vi "Check Tag WarnNSEstop Threshold.vi"(0 "Tick Counts Since Last Over Threshold":T4(array[cluster]), 1 "Warn/NS/Estop (0/1/2)":i32, 5 "Current Tick Count":u32, 7 "Tag from APU Setup File":string, 9 "Row of Tag/Warn/NS/Estop Vals":dbl[](array[numeric]), 11 "error in (no error)":errorcluster, 12 "Parsed Tags in":T2, 13 "Threshold Type (Neither/Max/Min)":enum16{"Neither", "Max", "Min"}(ring)) -> (4 "Tick Counts Since Last Over Threshold out":T4(array[cluster]), 8 "Alert":bool, 10 "Tag Thresh Info":T1, 15 "error out":errorcluster)   [LabVIEW 2018, in "RT - Analysis.lvlib"]
uses:
  RT - Analysis.lvlib
  Private Controls/Parsed Data Arrays.ctl
  Top Level/Shared Controls/Parsed Tag Cluster.ctl
  Public Controls/Alert Data.ctl
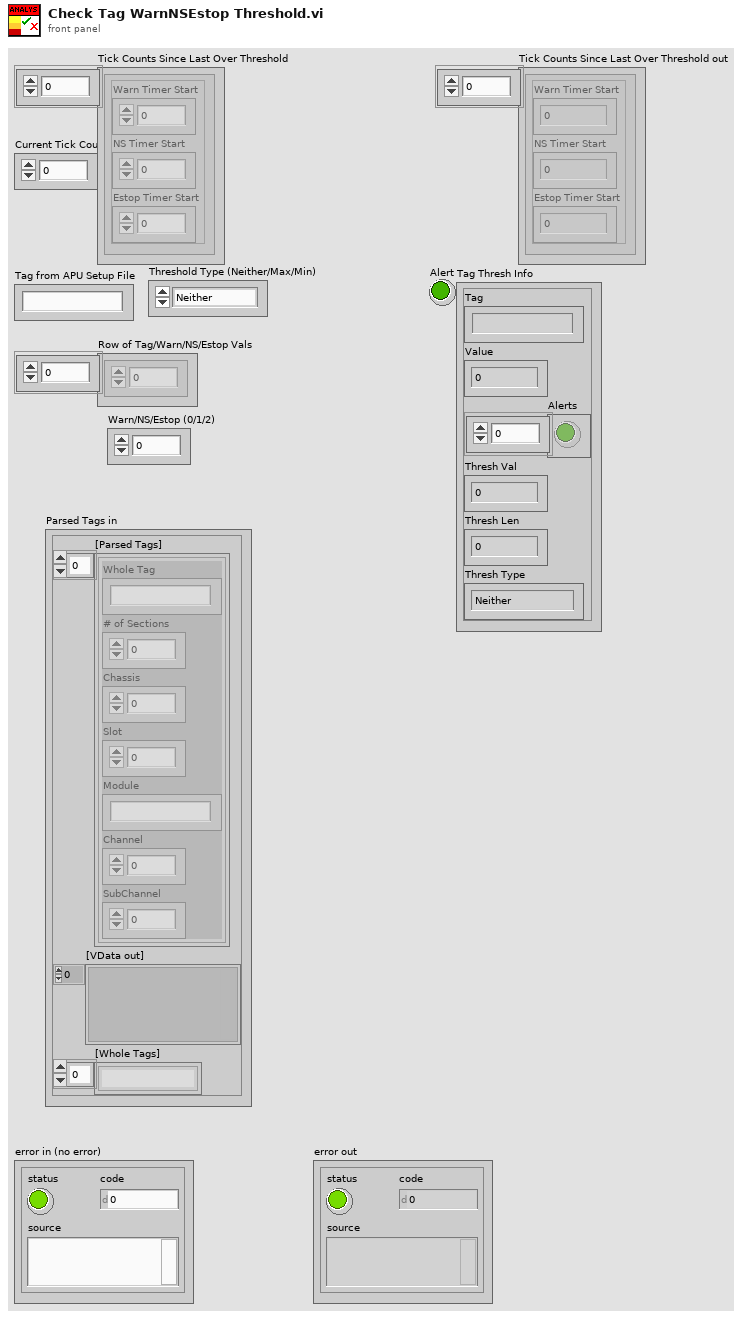
[diagram p1: front panel]
types:
  T1 = typedef "RT - Analysis.lvlib/Alert Data.ctl" = cluster{"Tag":string, "Value":dbl, "Alerts":bool[], "Thresh Val":dbl, "Thresh Len":dbl, "Thresh Type":enum16{"Neither", "Max", "Min"}}
  T2 = typedef "RT - Analysis.lvlib/Parsed Data Arrays.ctl" = cluster{"[Parsed Tags]":T3[], "[VData out]":variant[], "[Whole Tags]":string[]}
  T3 = typedef "Parsed Tag Cluster.ctl" = cluster{"Whole Tag":string, "# of Sections":u8, "Chassis":u8, "Slot":u8, "Module":string, "Channel":u8, "SubChannel":u8}
  T4 = cluster{"Warn Timer Start":u32, "NS Timer Start":u32, "Estop Timer Start":u32}[]
  T5 = cluster{"Warn Timer Start":u32, "NS Timer Start":u32, "Estop Timer Start":u32}
  T6 = cluster{"Warn Timer Start":u32, "Warn Timer Start":u32, "Warn Timer Start":u32}
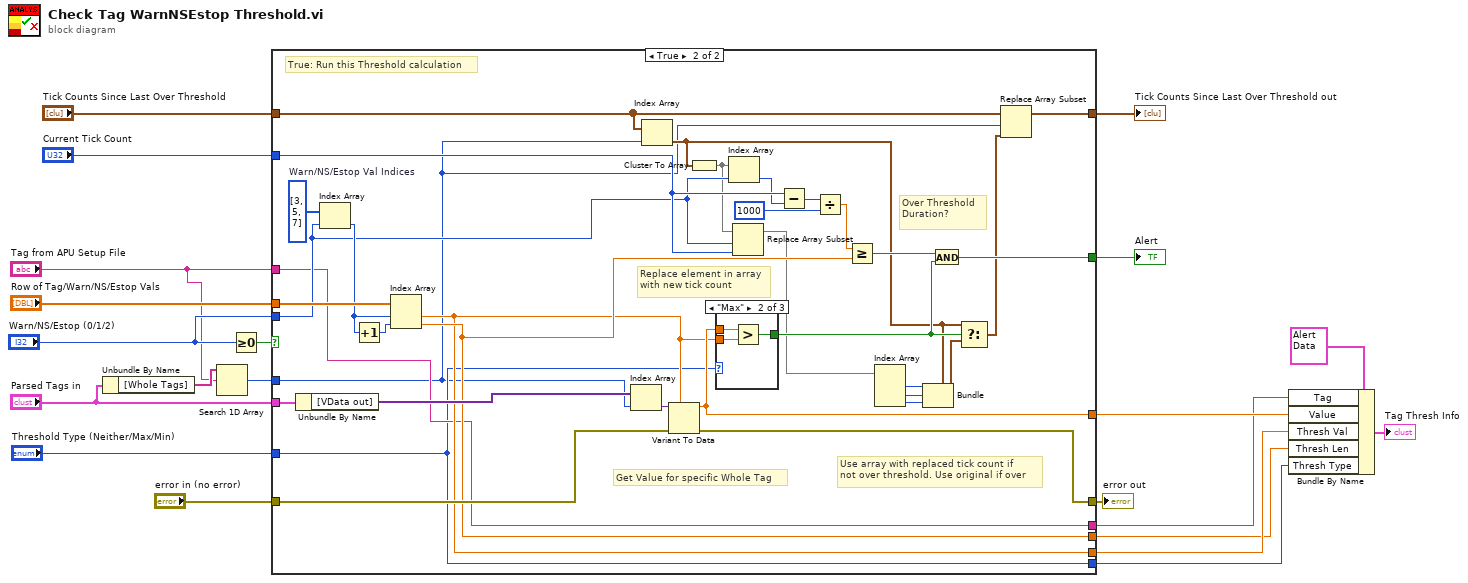
[diagram p0: block diagram]
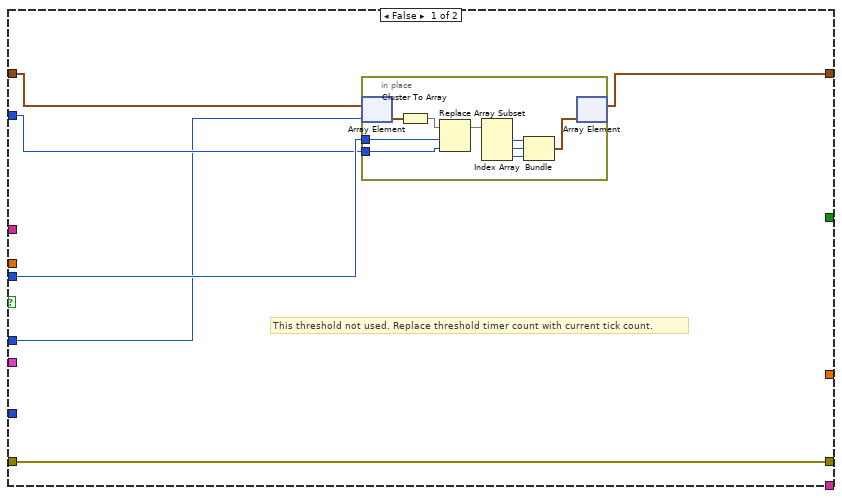
[diagram p2: hidden frame]
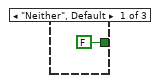
[diagram p3: hidden frame]
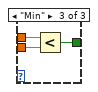
[diagram p4: hidden frame]
diagram:
  n1 = Unbundle By Name("Parsed Tags in") -> ("[Whole Tags]"=w3:string[])
  n2 = Search 1D Array(1D array=w3, element="Tag from APU Setup File") -> (index of element=w1:i32)  [unwired: 1 in]
  n3 = Greater Or Equal To 0?(x="Warn/NS/Estop (0/1/2)") -> (x >= 0?=w15:bool)
  n4 = case shown="True" w15 {
    tunnel: "Row of Tag/Warn/NS/Estop Vals" -> [_ w69]
    tunnel: "Tag from APU Setup File" -> [_ w54]
    tunnel: "error in (no error)" -> [w27 w64]
    tunnel: [w27 w63] -> w18
    tunnel: "Parsed Tags in" -> [_ w68]
    tunnel: "Tick Counts Since Last Over Threshold" -> [w24 w65]
    tunnel: [w22 w66] -> w20
    tunnel: "Current Tick Count" -> [w25 w62]
    tunnel: "Warn/NS/Estop (0/1/2)" -> [w26 w59]
    tunnel: [_ w58] -> w13
    tunnel: "Threshold Type (Neither/Max/Min)" -> [_ w53]
    tunnel: [_ w57] -> w10
    tunnel: [_ w56] -> w7
    tunnel: [_ w55] -> w8
    tunnel: [_ w54] -> w9
    tunnel: [_ w53] -> w6
    tunnel: w1 -> [w23 w37]
    frame False {
      # "This threshold not used. Replace threshold timer count with current tick count."
      n5 = in-place {
        in-place-border: w26 -> [w32]
        in-place-border: w25 -> [w31]
        n6 = in-place-array #1(w24, w23) -> (w29:T5)
        n7 = Cluster To Array(cluster=w29) -> (array=w33:u32[])
        n8 = Replace Array Subset(array=w33, new element=w31, index=w32) -> (w30:u32[])
        n9 = Index Array(array=w30) -> (element #1=w34:u32, element #2=w35:u32, element #3=w36:u32)  [unwired: 3 in]
        n10 = Bundle("Warn Timer Start"=w34, "Warn Timer Start"=w35, "Warn Timer Start"=w36) -> (w28:T6)  [unwired: 1 in]
        n11 = in-place-array #1(w28) -> (w22:T4)  [unwired: 1 out]
      }
    }
    frame True {
      w61 = i32[] [3, 5, 7]  # Warn/NS/Estop Val Indices
      # "Use array with replaced tick count if\nnot over threshold. Use original if over"
      # "Replace element in array\nwith new tick count"
      # "Over Threshold Duration?"
      # "Get Value for specific Whole Tag"
      # "True: Run this Threshold calculation"
      n12 = Unbundle By Name(w68) -> ("[VData out]"=w67:variant[])
      n13 = Index Array(array=w61, index=w59) -> (element=w60:i32)
      n14 = Increment(x=w60) -> (x+1=w70:i32)
      n15 = Index Array(array=w69, index #1=w60, index #2=w70) -> (element #1=w55:dbl, element #2=w56:dbl)
      n16 = Index Array(array=w67, index=w37) -> (element=w52:variant)
      n17 = Index Array(array=w65, index=w37) -> (element=w44:T5)
      n18 = Variant To Data(error in=w64, type=w55, Variant=w52) -> (data=w57:dbl, error out=w63:errorcluster)
      n19 = Cluster To Array(cluster=w44) -> (array=w42:u32[])
      n20 = case shown="\"Max\"" w53 {
        tunnel: w55 -> [_ w74 w77]
        tunnel: [FALSE w73 w76] -> w46
        tunnel: w57 -> [_ w72 w75]
        frame "Neither", Default {
        }
        frame "Max" {
          n21 = Greater?(x=w72, y=w74) -> (0:w73:bool)
        }
        frame "Min" {
          n22 = Less?(x=w75, y=w77) -> (x < y?=w76:bool)
        }
      }
      n23 = Index Array(array=w42, index=w59) -> (element=w50:u32)
      n24 = Replace Array Subset(array=w42, new element=w62, index=w59) -> (w38:u32[])
      n25 = Subtract(x=w62, y=w50) -> (x-y=w49:u32)
      n26 = Divide(x=w49, y=u32 1000) -> (x/y=w47:dbl)
      n27 = Greater Or Equal?(x=w47, y=w56) -> (x >= y?=w45:bool)
      n28 = Index Array(array=w38) -> (element #1=w41:u32, element #2=w40:u32, element #3=w39:u32)  [unwired: 3 in]
      n29 = Bundle(cluster=w44, "Warn Timer Start"=w41, "NS Timer Start"=w40, "Estop Timer Start"=w39) -> (w43:T5)
      n30 = And(x=w45, y=w46) -> (x .and. y?=w58:bool)
      n31 = Select(t=w44, s=w46, f=w43) -> (s? t:f=w51:T5)
      n32 = Replace Array Subset(array=w65, new element=w51, index=w37) -> (w66:T4)
    }
  }
  "Tick Counts Since Last Over Threshold out" <- w20
  "error out" <- w18
  "Alert" <- w13
  n33 = Bundle By Name(cluster=T1 {"Tag"="", "Value"=0.0, "Alerts"=[], "Thresh Val"=0.0, "Thresh Len"=0.0, "Thresh Type"=enum."Neither"} ("output cluster"), "Tag"=w9, "Value"=w10, "Thresh Val"=w8, "Thresh Len"=w7, "Thresh Type"=w6) -> (→"Tag Thresh Info":T1)
